vi "Pane Relief UI.vi"(8 "Error In":errorcluster, 11 "QD Launch VI Ref":refnum<vi>) -> (0 "Error Out":errorcluster)   [LabVIEW 2018]
uses:
  <resource>/dialog/QuickDrop/plugins/PaneRelief/Typedefs/Scrollbar Visibility--Enum.ctl
  <resource>/dialog/QuickDrop/plugins/PaneRelief/Typedefs/Splitter Sizing--Enum.ctl
  <resource>/dialog/QuickDrop/plugins/PaneRelief/Typedefs/Point--Cluster.ctl
  <resource>/dialog/QuickDrop/plugins/PaneRelief/Typedefs/UI Selections--Cluster.ctl
  <vilib>/Utility/sysdir.llb/System Directory Type.ctl
  <resource>/dialog/QuickDrop/plugins/PaneRelief/Classes/Splitter/Splitter.lvclass
  <resource>/dialog/QuickDrop/plugins/PaneRelief/Classes/Pane/Pane.lvclass
  <vilib>/Utility/miscctls.llb/LVRectTypeDef.ctl
  <resource>/dialog/QuickDrop/plugins/PaneRelief/Typedefs/Selection Colors--Cluster.ctl
panel:
  out "Nav Pic":picture
  in  "Label":string
  in  "Apply All - Scrollbar":bool
  in  "Apply All - Locked":bool
  in  "Apply All - Color":bool
  in  "Position":i32
  in  "Color":u32(colorbox)
  in  "Locked":bool
  in  "Sizing":T1
  in  "Vertical Scroll":T2
  in  "Horizontal Scroll":T2 caption="Scrollbar"
  in  "Origin":T3
  in  "Min Pane Size":T3
  # "Apply To All"
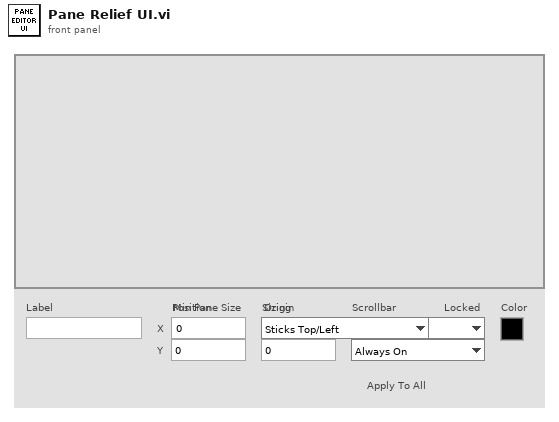
[diagram p1: front panel]
types:
  T1 = typedef "Splitter Sizing--Enum.ctl" = enum16{"Sticks Top/Left", "Sticks Bottom/Right", "Proportional"}
  T2 = typedef "Scrollbar Visibility--Enum.ctl" = enum16{"Always On", "Always Off", "Off While Running"}
  T3 = typedef "Point--Cluster.ctl" = cluster{"Horizontal":i32, "Vertical":i32}
  T4 = enum32{"Invalid", "Standard", "Closed", "Hidden", "Minimized", "Maximized"}
  T5 = enum32{"invalid app kind", "Development System", "Run Time System", "Student Edition", "Embedded LabVIEW", "Evaluation", "Custom"}
  T6 = enum16{"open", "replace", "create", "open or create", "replace or create", "replace or create with confirmation"}
  T7 = typedef "LVRectTypeDef.ctl" = cluster{"Left":i16, "Top":i16, "Right":i16, "Bottom":i16}
  T8 = typedef "LVPoint32TypeDef.ctl" = cluster{"Horizontal":i32, "Vertical":i32}
  T9 = typedef "UI Selections--Cluster.ctl" = cluster{"Mouse-over Idx":i32, "Mouse-over Splitter? (F: Pane)":bool, "Selected Idx":i32, "Selected Splitter? (F: Pane)":bool}
  T10 = cluster{"Core":cluster{"Current VI Reference":refnum<vi>, "Close Panel on Exit?":bool}, "QD Launch VI Ref":refnum<vi>, "Splitters[]":refnum<class "Splitter.lvclass">[], "Panes[]":refnum<class "Pane.lvclass">[], "UI Selections":T9, "Scale Factor":dbl, "Nav Pic Offset":T3, "Persistent Data Folder":path, "Persistent Data File":string}
  T11 = typedef "System Directory Type.ctl" = i32
  T12 = cluster{"Current VI Reference":refnum<vi>, "Close Panel on Exit?":bool}
  T13 = typedef "LVBoundsTypeDef.ctl" = cluster{"Width":u32, "Height":u32}
  T14 = typedef "LVPointTypeDef.ctl" = cluster{"Horizontal":i16, "Vertical":i16}
  T15 = typedef "Selection Colors--Cluster.ctl" = cluster{"Normal":u32, "Mouse-over":u32, "Selected":u32}
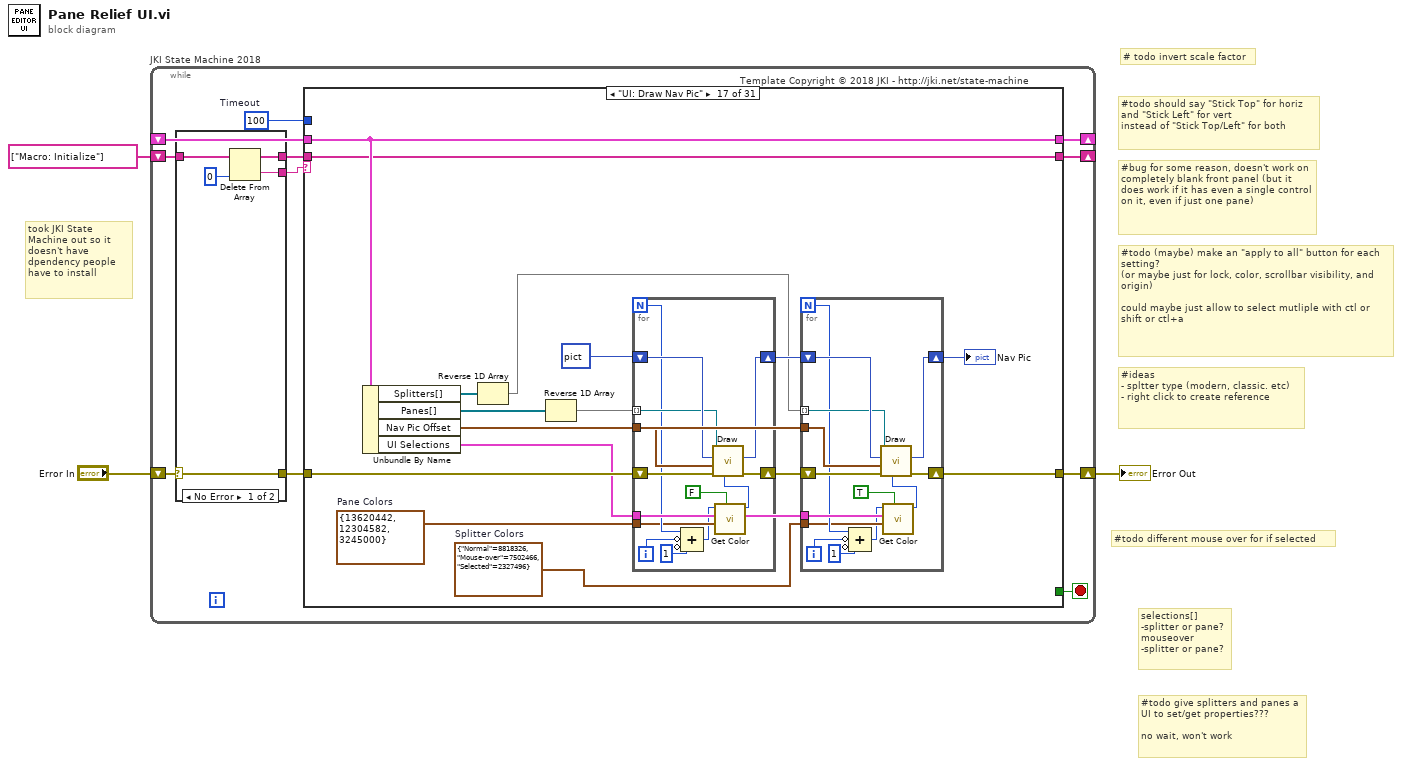
[diagram p0: block diagram]
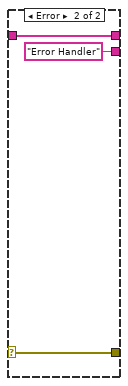
[diagram p2: hidden frame]
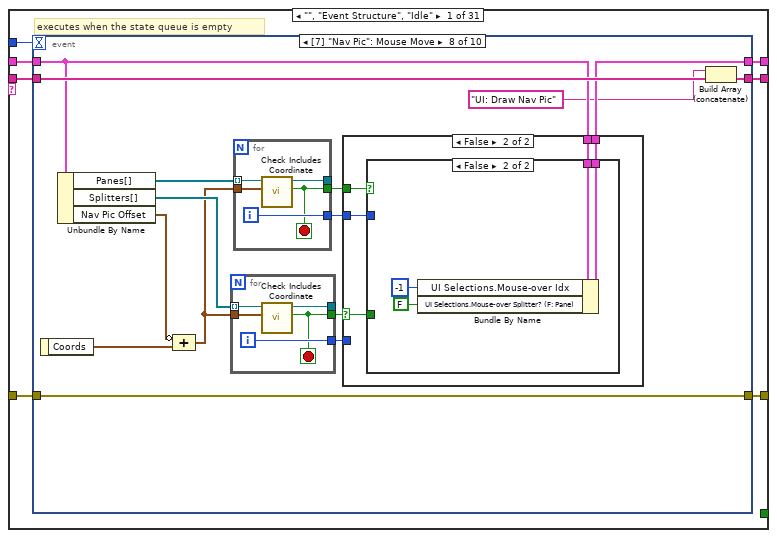
[diagram p3: hidden frame]
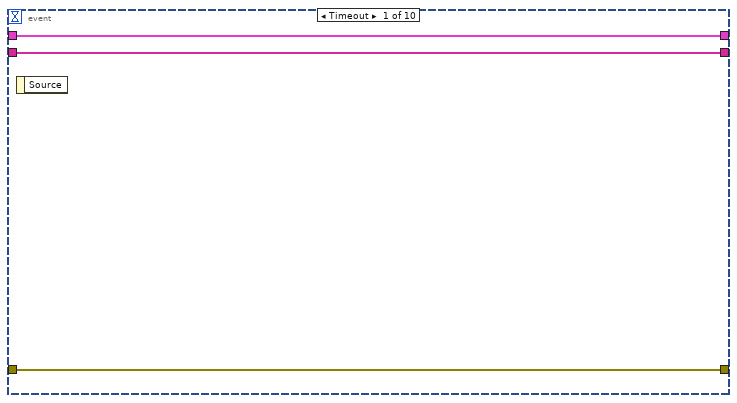
[diagram p4: hidden frame]
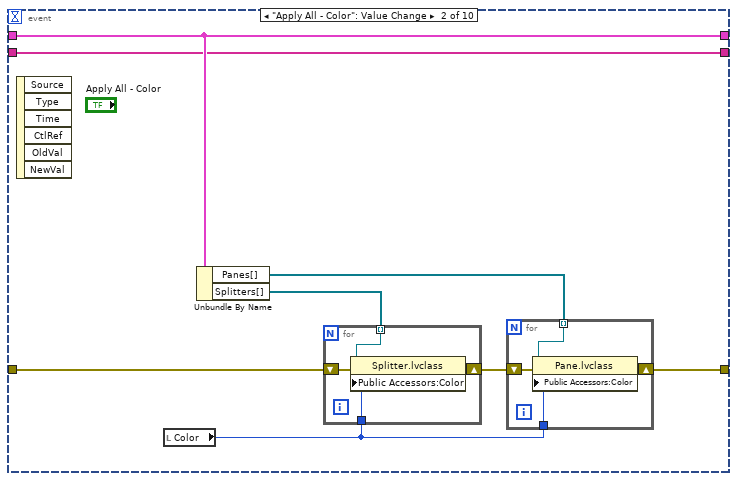
[diagram p5: hidden frame]
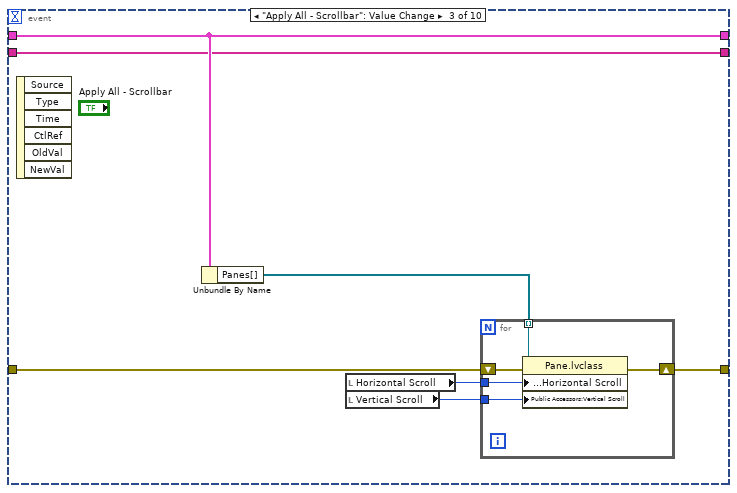
[diagram p6: hidden frame]
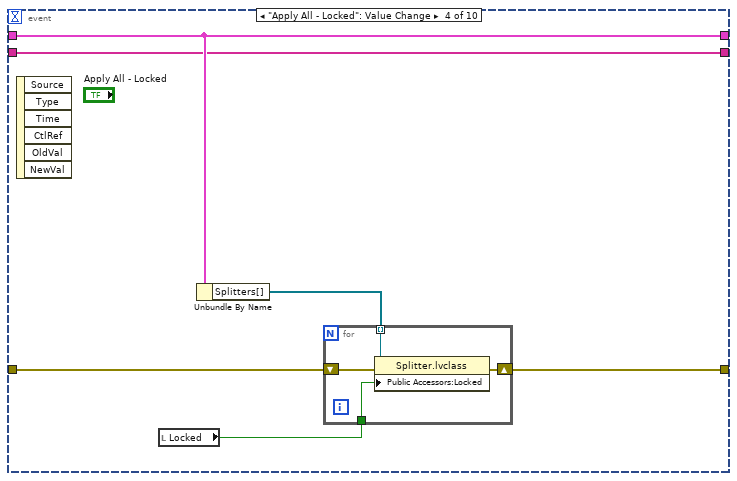
[diagram p7: hidden frame]
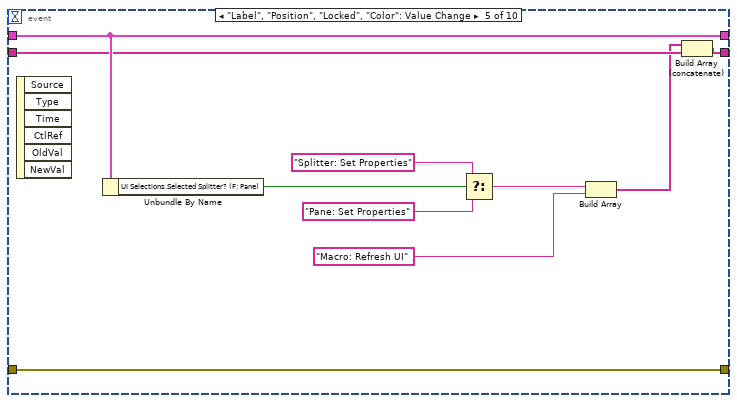
[diagram p8: hidden frame]
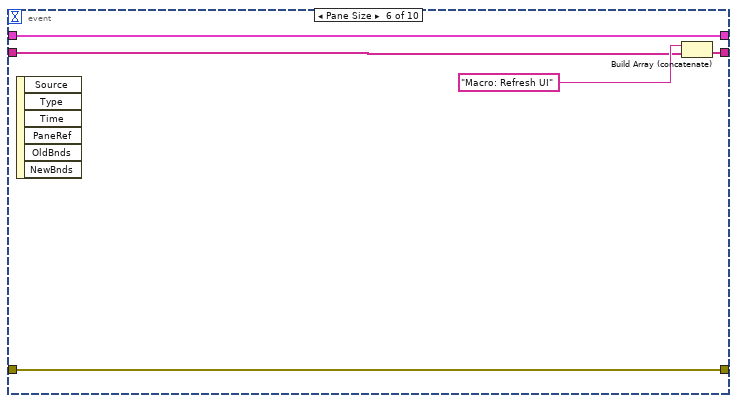
[diagram p9: hidden frame]
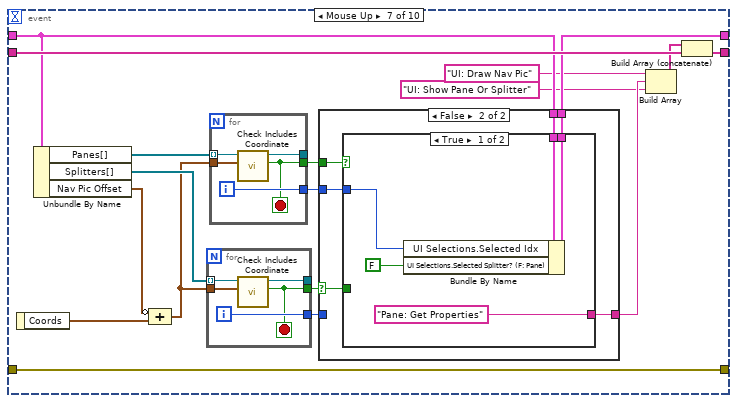
[diagram p10: hidden frame]
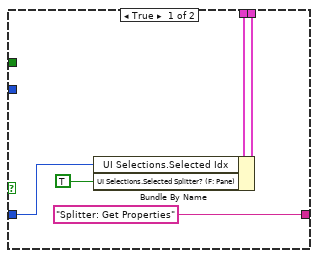
[diagram p11: hidden frame]
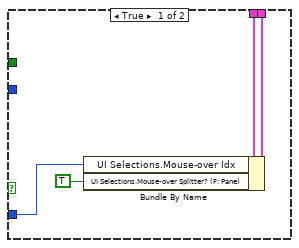
[diagram p13: hidden frame]
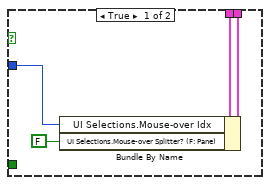
[diagram p14: hidden frame]
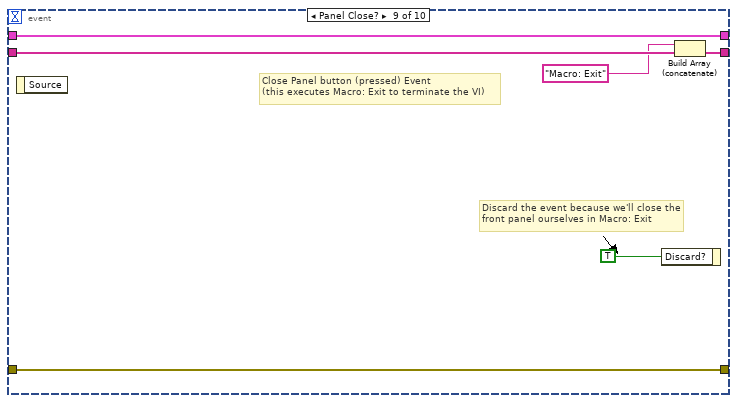
[diagram p15: hidden frame]
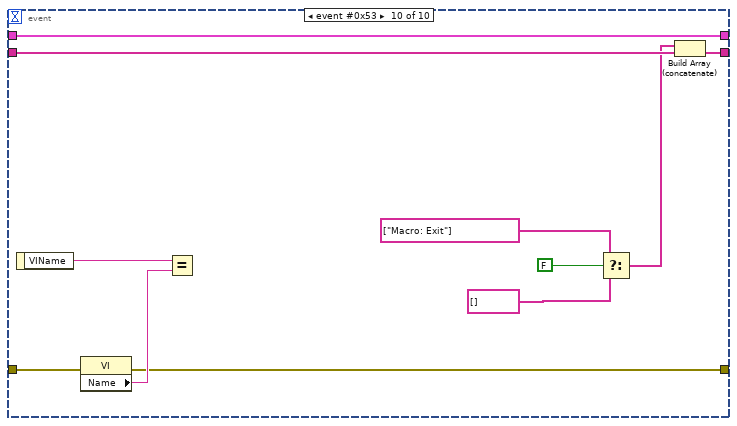
[diagram p16: hidden frame]
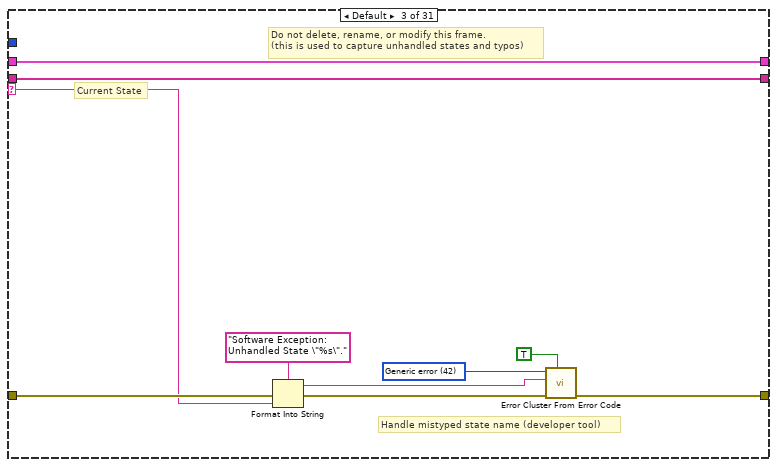
[diagram p18: hidden frame]
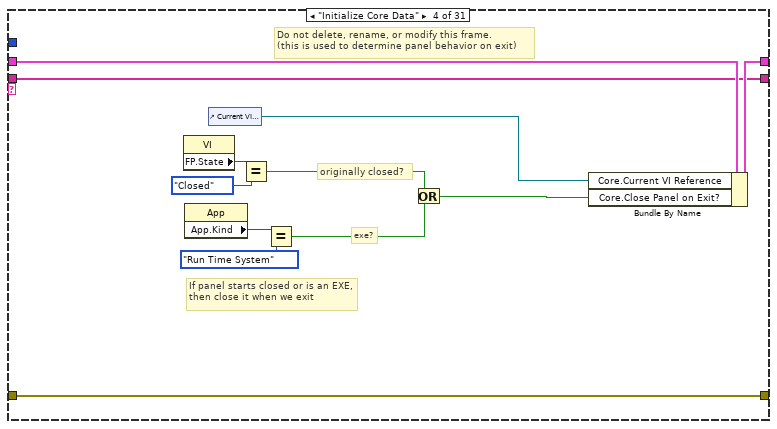
[diagram p19: hidden frame]
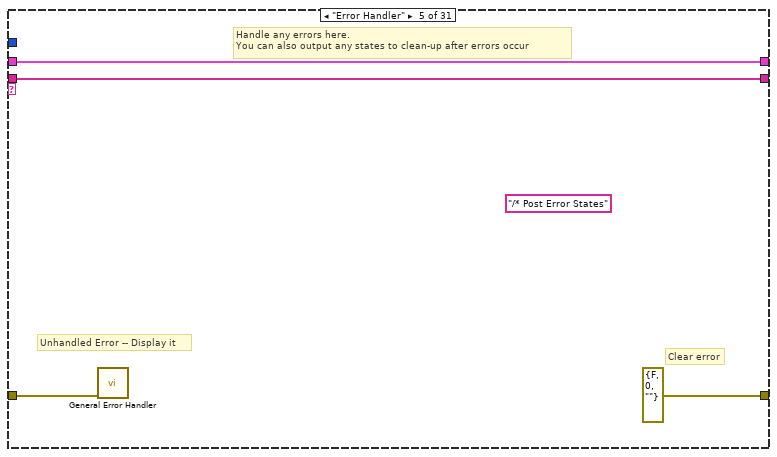
[diagram p20: hidden frame]
diagram:
  # "#todo give splitters and panes a UI to set/get properties???\n\nno wait, won't work"
  # "# todo invert scale factor"
  # "selections[]\n-splitter or pane?\nmouseover\n-splitter or pane?"
  # "#todo different mouse over for if selected"
  # "took JKI State Machine out so it doesn't have dpendency people have to install"
  # "#ideas\n- spltter type (modern, classic. etc)\n- right click to create reference"
  # "#todo (maybe) make an \"apply to all\" button for each setting?\n(or maybe just for lock, color, scrollbar visibility, and origin)\n\ncould maybe just allow to select mutliple with ctl or shift or ctl+a"
  # "#todo should say \"Stick Top\" for horiz and \"Stick Left\" for vert\ninstead of \"Stick Top/Left\" for both"
  # "#bug for some reason, doesn't work on completely blank front panel (but it does work if it has even a single control on it, even if just one pane)"
  n1 = while "JKI State Machine 2018" {
    shift-right: [w11] -> _
    shift-left: _ -> [w10]
    shift-right: [w14] -> w2
    shift-left: "Error In" -> [w4]
    shift-right: [w13] -> _
    shift-left: string[] ["Macro: Initialize"] -> [w8]
    stop <- w12 stop-if-true
    w9 = 100  # Timeout
    # "Template Copyright © 2018 JKI - http://jki.net/state-machine"
    n2 = case shown="No Error" w4 {
      selector: w4 -> [w15 w22]
      tunnel: w8 -> [w19 w21]
      tunnel: [w18 w21] -> w7
      tunnel: [w17 "Error Handler" ("String")] -> w6
      tunnel: [w15 w22] -> w5
      frame No Error {
        n3 = Delete From Array(array=w19, index=0) -> (deleted portion=w17:string, array with subset deleted=w18:string[])  [unwired: 1 in]
      }
      frame Error {
      }
    }
    n4 = case shown="\"UI: Draw Nav Pic\"" w6 {
      selector: w6 -> [_ _ w196 _ _ _ _ _ _ _ _ _ _ _ _ _ _ _ _ _ _ _ _ _ _ _ _ _ _ _ _]
      tunnel: w7 -> [w29 w190 w193 w203 w215 w219 w223 w228 w243 w248 w251 w254 w286 w311 w319 w347 w382 w412 w416 w425 w441 w450 w455 w460 w466 w473 w477 w488 w500 w503 w516]
      tunnel: w10 -> [w27 w191 w197 w209 w217 w222 w224 _ w244 w249 w253 w257 w299 w318 w326 w351 w383 w415 w419 w427 w443 w451 w456 w461 w471 w474 w487 w499 w501 w515 w528]
      tunnel: [w26 w192 w199 w213 errorcluster {"status"=FALSE, "code"=0, "source"=""} ("error out") w221 w225 w241 w245 w250 w252 w259 w287 w317 w323 w350 w374 w413 w417 w428 w444 w452 w457 w462 w472 w475 w482 w494 w502 w510 w523] -> w14
      tunnel: w5 -> [w23 w192 w198 w213 w216 w221 w225 w241 w246 w250 w252 w279 w296 w317 w331 w353 w380 w414 w418 w429 w445 w452 w457 w462 w472 w475 w483 w495 w502 w511 w524]
      tunnel: [w28 w190 w193 w203 w215 w219 w223 w228 w243 w248 w251 w254 w286 w311 w319 w347 w382 w412 w416 w425 w441 w450 w453 w458 w465 w473 w477 w488 w500 w503 w516] -> w13
      tunnel: [_ _ _ _ _ TRUE _ _ _ _ _ _ _ _ _ _ _ _ _ _ _ _ _ _ _ _ _ _ _ _ _] -> w12
      tunnel: [w25 w191 w197 w214 w217 w222 w224 w242 w244 w249 w253 w257 w299 w318 w321 w352 w383 w415 w419 w427 w443 w451 w456 w461 w471 w474 w487 w499 w501 w515 w528] -> w11
      tunnel: w9 -> [w24 _ _ _ _ _ _ _ _ _ _ _ _ _ _ _ _ _ _ _ _ _ _ _ _ _ _ _ _ _ _]
      frame "", "Event Structure", "Idle" {
        # "executes when the state queue is empty"
        n5 = event shown="[7] \"Nav Pic\": Mouse Move" {
          selector: _ -> [_ _ _ _ _ _ _ _ _ _]
          dyn-events: _ -> [_ _ _ _ _ _ _ _ _ _]
          timeout: w24 -> [_ _ _ _ _ _ _ _ _ _]
          tunnel: w29 -> [w30 w33 w49 w61 w73 w82 w103 w145 w175 w188]
          tunnel: [w30 w33 w49 w61 w71 w81 w102 w144 w173 w187] -> w28
          tunnel: w27 -> [w31 w36 w54 w64 w77 w84 w99 w141 w177 w189]
          tunnel: [w32 w37 w55 w62 w80 w85 w101 w143 w178 w184] -> w26
          tunnel: [w31 w36 w54 w64 w77 w84 w100 w142 w177 w189] -> w25
          tunnel: w23 -> [w32 w40 w52 w66 w80 w85 w101 w143 w178 w183]
          event Timeout {
            n6 = event-data() -> ()  [unwired: 1 in, 1 out]
          }
          event "Apply All - Color": Value Change {
            n7 = event-data() -> ()  [unwired: 1 in, 6 out]
            n8 = local read "Color"() -> (w38:u32)
            n9 = Unbundle By Name(w36) -> ("Panes[]"=w34:refnum<class "Pane.lvclass">[], "Splitters[]"=w35:refnum<class "Splitter.lvclass">[])
            n10 = for {
              tunnel: w38 -> [w45]
              shift-right: [w47] -> w39
              shift-left: w40 -> [w48]
              tunnel: w35 -> [w46] mode=indexing
              n11 = property class="Splitter.lvclass"(reference=w46, error in=w48, "Public Accessors:Color"=w45) -> (error out=w47:errorcluster)  [unwired: 1 out]
            }
            n12 = for {
              tunnel: w38 -> [w43]
              shift-right: [w42] -> w37
              shift-left: w39 -> [w44]
              tunnel: w34 -> [w41] mode=indexing
              n13 = property class="Pane.lvclass"(reference=w41, error in=w44, "Public Accessors:Color"=w43) -> (error out=w42:errorcluster)  [unwired: 1 out]
            }
          }
          event "Apply All - Scrollbar": Value Change {
            n14 = event-data() -> ()  [unwired: 1 in, 6 out]
            n15 = Unbundle By Name(w54) -> ("Panes[]"=w53:refnum<class "Pane.lvclass">[])
            n16 = local read "Horizontal Scroll"() -> (w51:T2)
            n17 = local read "Vertical Scroll"() -> (w50:T2)
            n18 = for {
              shift-right: [w59] -> w55
              shift-left: w52 -> [w60]
              tunnel: w53 -> [w58] mode=indexing
              tunnel: w51 -> [w57]
              tunnel: w50 -> [w56]
              n19 = property class="Pane.lvclass"(reference=w58, error in=w60, "Public Accessors:Horizontal Scroll"=w57, "Public Accessors:Vertical Scroll"=w56) -> (error out=w59:errorcluster)  [unwired: 1 out]
            }
          }
          event "Apply All - Locked": Value Change {
            n20 = event-data() -> ()  [unwired: 1 in, 6 out]
            n21 = local read "Locked"() -> (w65:bool)
            n22 = Unbundle By Name(w64) -> ("Splitters[]"=w63:refnum<class "Splitter.lvclass">[])
            n23 = for {
              tunnel: w65 -> [w68]
              shift-right: [w69] -> w62
              shift-left: w66 -> [w70]
              tunnel: w63 -> [w67] mode=indexing
              n24 = property class="Splitter.lvclass"(reference=w67, error in=w70, "Public Accessors:Locked"=w68) -> (error out=w69:errorcluster)  [unwired: 1 out]
            }
          }
          event "Label", "Position", "Locked", "Color": Value Change {
            n25 = event-data() -> ()  [unwired: 1 in, 6 out]
            n26 = Unbundle By Name(w77) -> ("UI Selections.Selected Splitter? (F: Pane)"=w76:bool)
            n27 = Select(t="Splitter: Set Properties" ("State(s) in Front (\"\")"), s=w76, f="Pane: Set Properties" ("State(s) in Front (\"\")")) -> (s? t:f=w75:string)
            n28 = Build Array(w75, "Macro: Refresh UI" ("State(s) in Front (\"\")")) -> (w72:string[])
            n29 = Build Array (concatenate)(w72, w73) -> (w71:string[])
          }
          event Pane Size {
            n30 = event-data() -> ()  [unwired: 1 in, 6 out]
            n31 = Build Array (concatenate)("Macro: Refresh UI", w82) -> (w81:string[])
          }
          event Mouse Up {
            n32 = event-data() -> ("Coords"=w92:T8)  [unwired: 1 in]
            n33 = Unbundle By Name(w99) -> ("Panes[]"=w90:refnum<class "Pane.lvclass">[], "Splitters[]"=w89:refnum<class "Splitter.lvclass">[], "Nav Pic Offset"=w93:T3)
            n34 = Compound Arithmetic op=ADD(invert w93, w92) -> (w88:T3)
            n35 = for {
              tunnel: [w108] -> _
              tunnel: [w104] -> w98
              tunnel: w89 -> [w107] mode=indexing
              tunnel: w88 -> [w106]
              tunnel: [w105] -> w86
              i -> [w105]
              stop <- w104 stop-if-true
              n36 = call-dynamic "Check Includes Coordinate.vi"("Coordinate"=w106, "Panel Object in"=w107) -> ("Included?"=w104:bool, "Panel Object out"=w108:refnum<class "Splitter.lvclass">)  [unwired: 7 in, 1 out]
            }
            n37 = for {
              tunnel: [w109] -> w97
              tunnel: [w113] -> _
              tunnel: w90 -> [w112] mode=indexing
              tunnel: w88 -> [w111]
              tunnel: [w110] -> w87
              i -> [w110]
              stop <- w109 stop-if-true
              n38 = call-dynamic "Check Includes Coordinate.vi"("Coordinate"=w111, "Panel Object in"=w112) -> ("Included?"=w109:bool, "Panel Object out"=w113:refnum<class "Pane.lvclass">)  [unwired: 7 in, 1 out]
            }
            n39 = case shown="False" w98 {
              selector: w98 -> [_ w122]
              tunnel: [w118 w124] -> w100
              tunnel: w99 -> [w117 w123]
              tunnel: w97 -> [_ w121]
              tunnel: ["Splitter: Get Properties" w120] -> w96
              tunnel: w87 -> [_ w119]
              tunnel: w86 -> [w114 _]
              frame True {
                n40 = Bundle By Name(cluster=w117, "UI Selections.Selected Idx"=w114, "UI Selections.Selected Splitter? (F: Pane)"=TRUE ("UI Selections.Splitter? (F: Pane)")) -> (w118:T10)
              }
              frame False {
                n41 = case shown="True" w121 {
                  tunnel: [w129 w130] -> w124
                  tunnel: w123 -> [w128 w130]
                  tunnel: w122 -> [_ _]
                  tunnel: ["Pane: Get Properties" _] -> w120
                  tunnel: w119 -> [w125 _]
                  frame True {
                    n42 = Bundle By Name(cluster=w128, "UI Selections.Selected Idx"=w125, "UI Selections.Selected Splitter? (F: Pane)"=FALSE ("UI Selections.Splitter? (F: Pane)")) -> (w129:T10)
                  }
                  frame False {
                  }
                }
              }
            }
            n43 = Build Array("UI: Draw Nav Pic", w96, "UI: Show Pane Or Splitter") -> (w94:string[])
            n44 = Build Array (concatenate)(w94, w103) -> (w102:string[])
          }
          event "Nav Pic": Mouse Move {
            n45 = event-data() -> ("Coords"=w137:T8)  [unwired: 1 in]
            n46 = Unbundle By Name(w141) -> ("Panes[]"=w136:refnum<class "Pane.lvclass">[], "Splitters[]"=w135:refnum<class "Splitter.lvclass">[], "Nav Pic Offset"=w138:T3)
            n47 = Compound Arithmetic op=ADD(invert w138, w137) -> (w134:T3)
            n48 = for {
              tunnel: [w150] -> _
              tunnel: [w146] -> w140
              tunnel: w135 -> [w149] mode=indexing
              tunnel: w134 -> [w148]
              tunnel: [w147] -> w132
              i -> [w147]
              stop <- w146 stop-if-true
              n49 = call-dynamic "Check Includes Coordinate.vi"("Coordinate"=w148, "Panel Object in"=w149) -> ("Included?"=w146:bool, "Panel Object out"=w150:refnum<class "Splitter.lvclass">)  [unwired: 7 in, 1 out]
            }
            n50 = for {
              tunnel: [w151] -> w139
              tunnel: [w155] -> _
              tunnel: w136 -> [w154] mode=indexing
              tunnel: w134 -> [w153]
              tunnel: [w152] -> w133
              i -> [w152]
              stop <- w151 stop-if-true
              n51 = call-dynamic "Check Includes Coordinate.vi"("Coordinate"=w153, "Panel Object in"=w154) -> ("Included?"=w151:bool, "Panel Object out"=w155:refnum<class "Pane.lvclass">)  [unwired: 7 in, 1 out]
            }
            n52 = case shown="False" w140 {
              selector: w140 -> [_ w162]
              tunnel: [w159 w164] -> w142
              tunnel: w141 -> [w158 w163]
              tunnel: w139 -> [_ w161]
              tunnel: w133 -> [_ w160]
              tunnel: w132 -> [w156 _]
              frame True {
                n53 = Bundle By Name(cluster=w158, "UI Selections.Mouse-over Idx"=w156, "UI Selections.Mouse-over Splitter? (F: Pane)"=TRUE ("UI Selections.Splitter? (F: Pane)")) -> (w159:T10)
              }
              frame False {
                n54 = case shown="False" w161 {
                  tunnel: [w168 w169] -> w164
                  tunnel: w163 -> [w167 w170]
                  tunnel: w162 -> [_ _]
                  tunnel: w160 -> [w165 _]
                  frame True {
                    n55 = Bundle By Name(cluster=w167, "UI Selections.Mouse-over Idx"=w165, "UI Selections.Mouse-over Splitter? (F: Pane)"=FALSE ("UI Selections.Splitter? (F: Pane)")) -> (w168:T10)
                  }
                  frame False {
                    n56 = Bundle By Name(cluster=w170, "UI Selections.Mouse-over Idx"=-1, "UI Selections.Mouse-over Splitter? (F: Pane)"=FALSE ("UI Selections.Splitter? (F: Pane)")) -> (w169:T10)
                  }
                }
              }
            }
            n57 = Build Array (concatenate)("UI: Draw Nav Pic", w145) -> (w144:string[])
          }
          event Panel Close? {
            # "Discard the event because we'll close the front panel ourselves in Macro: Exit"
            # "Close Panel button (pressed) Event\n(this executes Macro: Exit to terminate the VI)"
            n58 = event-data() -> ()  [unwired: 1 in, 1 out]
            n59 = event-data("Discard?"=TRUE) -> ()  [unwired: 1 in, 1 out]
            n60 = Build Array (concatenate)("Macro: Exit", w175) -> (w173:string[])
          }
          event event #0x53 {
            n61 = event-data() -> ("VIName"=w186:string)  [unwired: 1 in]
            n62 = property class="VI"(error in=w183) -> (error out=w184:errorcluster, "Name"=w185:string)  [unwired: 1 in, 1 out]
            n63 = Equal?(x=w186, y=w185) -> ()  [unwired: 1 out]
            n64 = Select(t=string[] ["Macro: Exit"], s=FALSE, f=string[] []) -> (s? t:f=w180:string[])
            n65 = Build Array (concatenate)(w180, w188) -> (w187:string[])
          }
        }
      }
      frame "---------- Core ----------" {
        # "Do not put any code in this frame.\n(it is a separator no-op)"
      }
      frame Default {
        w195 = 42 items=["No error", "Argument error", "Memory is full", "Out of zone", "End of file", "File already open", "Generic file I/O error", "File not found", "File permission error", "Disk is full", "Duplicate path", "Too many files open", "System feature not enabled", "Resource file not found", "Cannot add resource", "Resource not found", "Image not found", "Image memory error", "Pen does not exist", "Config type invalid", "Config token not found", "Config parse error", "Config memory error", "Bad external code format", "Bad external code offset", "External code not present", "Null window", "Destroy window error", "Null menu", "Print aborted", "Bad print record", "Print driver error", "Windows error during printing", "Memory error during printing", "Print dialog error", "Generic print error", "Invalid device refnum", "Device not found", "Device parameter error", "Device unit error", "Cannot open device", "Device call aborted", "Generic error", "Cancelled by user", "Object ID too low", "Object ID too high", "Object not in heap", "Unknown heap", "Unknown object (invalid DefProc)", "Unknown object (DefProc not in table)", "Message out of range", "Invalid (null) method", "Unknown message", "Manager call not supported", "Bad address", "Network operation in progress", "Network operation timed out", "Connection is busy", "Network attribute not supported", "Network error", "Address in use", "System out of memory", "Connection aborted", "Connection refused", "Not connected", "Already connected", "Connection closed", "Initialization error (interapplication manager)", "Bad occurrence", "Wait on unbound occurrence handler", "Occurrence queue overflow", "Datalog type conflict", "Unused", "Unrecognized type (interapplication manager)", "Memory corrupt", "Failed to make temporary DLL", "Old CIN version", "Drag socket not found", "Failed to load drop-object", "Failed to register OLE object", "Failed to release OLE object", "Format specifier type mismatch", "Unknown format specifier", "Too few format specifiers", "Too many format specifiers", "Scan failed", "Newer CIN version", "Error converting to variant", "Runtime menu error", "Password tampered", "Variant attribute not found", "Incompatible variant data type", "Event data is not available", "Event Store is not present", "Occurrence is not found", "Event Queue is not created", "Event info is not available", "Refnum passed is NULL", "Error retrieving Class GUID", "Error retrieving CoClass GUID", "Error retrieving TypeLib GUID.", "Bad built application magic bytes.", "Specific driver is different from the specific driver associated with the Logical Name.", "There is no session opened to the class driver.", "Max Error", "MAX - Error with config objects", "MAX - Error loading configuration", "MAX - Group not supported"]
        # "Current State"
        # "Do not delete, rename, or modify this frame.\n(this is used to capture unhandled states and typos)"
        # "Handle mistyped state name (developer tool)"
        n66 = Format Into String(format string="Software Exception: Unhandled State \"%s\"." ("message"), error in=w198, w196) -> (resulting string=w201:string, error out=w200:errorcluster)  [unwired: 1 in]
        n67 = call <vilib>:"Error Cluster From Error Code.vi"("show call chain? (False)"=TRUE, "error in (no error)"=w200, "error message (\"\")"=w201, "error code (0)"=w195) -> ("error out"=w199:errorcluster)  [unwired: 5 in]
      }
      frame "Initialize Core Data" {
        # "Do not delete, rename, or modify this frame.\n(this is used to determine panel behavior on exit)"
        # "originally closed?"
        # "exe?"
        # "If panel starts closed or is an EXE, then close it when we exit"
        n68 = property class="VI"() -> ("FP.State"=w206:T4)  [unwired: 2 in, 2 out]
        n69 = property class="App"() -> ("App.Kind"=w212:T5)  [unwired: 2 in, 2 out]
        n70 = control-ref of="Current VI Reference"() -> (w207:refnum<vi>)
        n71 = Equal?(x=w206, y=T4."Closed" ("Front Panel Window:State")) -> (x = y?=w204:bool)
        n72 = Equal?(x=w212, y=T5."Run Time System" ("Application:Kind")) -> (x = y?=w210:bool)
        n73 = Or(x=w204, y=w210) -> (x .or. y?=w208:bool)
        n74 = Bundle By Name(cluster=w209, "Core.Current VI Reference"=w207, "Core.Close Panel on Exit?"=w208) -> (w214:T10)
      }
      frame "Error Handler" {
        (unwired) "/* Post Error States"
        # "Unhandled Error -- Display it"
        # "Handle any errors here.\nYou can also output any states to clean-up after errors occur"
        # "Clear error"
        n75 = call <vilib>:"General Error Handler.vi"("error in (no error)"=w216) -> ()  [unwired: 10 in, 5 out]
      }
      frame "Exit" {
        # "Do not put any code in this frame.\n(No errors that occur here will be handled.)"
      }
      frame "---------- Data ----------" {
        # "Do not put any code in this frame.\n(It is a separator no-op. You can make a copy of this frame to create a new Data frame)"
      }
      frame "Data: Initialize" {
        w226 = refnum<class "Pane.lvclass">[] []  # Panes[]
        w227 = refnum<class "Splitter.lvclass">[] []  # Splitters[]
        w232 = path ""  # Persistent Data Folder
        w229 = "PaneReliefPersistentData.txt"  # Persistent Data File
        w235 = T11 3 items=["User Home"=0, "User Desktop"=1, "User Documents"=2, "User Application Data"=3, "User Preferences"=4, "User Temporary"=5, "Public Documents"=6, "Public Application Data"=7, "Public Preferences"=8, "Public Cache"=13, "System Core Libraries"=9, "System Installed Libraries"=10, "Application Files"=11, "Boot Volume Root"=12] ("system directory type")
        w236 = T3 {"Horizontal"=0, "Vertical"=0}  # Nav Pic Offset
        w237 = 0.0  # Scale Factor
        w238 = T9 {"Mouse-over Idx"=-1, "Mouse-over Splitter? (F: Pane)"=FALSE, "Selected Idx"=0, "Selected Splitter? (F: Pane)"=FALSE}  # UI Selections
        w239 = T12 {"Current VI Reference"=refnum, "Close Panel on Exit?"=FALSE}  # Core
        # "Data names and types of shift register data are defined by this bundle."
        # "Initialize the shift-register data, here.\n(data names are defined by what you wire into the bundle function)"
        n76 = call <vilib>:"Get System Directory.vi"("system directory type"=w235) -> ("system directory"=w233:path)  [unwired: 10 in]
        n77 = Build Path(base path=w233, name or relative path="PaneRelief") -> (appended path=w230:path)
        n78 = Variant To Data(type=w232, Variant=w230) -> (data=w231:path)  [unwired: 1 in, 1 out]
        n79 = Bundle("Core"=w239, "QD Launch VI Ref"="QD Launch VI Ref", "Splitters[]"=w227, "Panes[]"=w226, "UI Selections"=w238, "Scale Factor"=w237, "Nav Pic Offset"=w236, "Persistent Data Folder"=w231, "Persistent Data File"=w229) -> (w242:T10)  [unwired: 1 in]
      }
      frame "Data: Cleanup" {
        # "Cleanup any data and references, here.\n(this is called automatically, by the Macro: Exit)"
        n80 = Unbundle By Name(w244) -> ("Core.Current VI Reference"=w247:refnum<vi>)
        n81 = Close Reference(reference=w247, error in (no error)=w246) -> (error out=w245:errorcluster)
      }
      frame "---------- UI ----------" {
        # "Do not put any code in this frame.\n(It is a separator no-op. You can make a copy of this frame to create a new UI frame)"
      }
      frame "UI: Initialize" {
        # "Initialize the User Interface, here.\n(this is called automatically, by the Macro: Init)"
      }
      frame "UI: Save Window Bounds" {
        n82 = property class="VI"(error in=w279) -> (error out=w278:errorcluster, "Front Panel.WinBounds"=w263:T7)  [unwired: 1 in, 1 out]
        n83 = Unbundle By Name(w257) -> ("Persistent Data Folder"=w256:path, "Persistent Data File"=w255:string)
        n84 = Unbundle By Name(w263) -> ("Left"=w268:i16, "Top"=w266:i16, "Right"=w265:i16, "Bottom"=w264:i16)
        n85 = Format Into String(format string="%d,%d,%d,%d", error in=w278, w268, w266, w265, w264) -> (resulting string=w262:string, error out=w269:errorcluster)  [unwired: 1 in]
        n86 = call <vilib>:"Check if File or Folder Exists.vi"("error in (no error)"=w269, "path"=w256) -> ("error out"=w277:errorcluster, "file or folder exists?"=w276:bool, "dup path"=w275:path)  [unwired: 7 in]
        n87 = case shown="False" w276 {
          tunnel: w277 -> [w283 w284]
          tunnel: w275 -> [w282 w285]
          tunnel: [w281 w285] -> w273
          tunnel: [w280 w284] -> w271
          frame False {
            n88 = Create Folder(path (use dialog)=w282, error in=w283) -> (created path=w281:path, error out=w280:errorcluster)  [unwired: 1 in, 1 out]
          }
          frame True {
          }
        }
        n89 = Build Path(base path=w273, name or relative path=w255) -> (appended path=w272:path)
        n90 = Open/Create/Replace File(file path (use dialog)=w272, error in=w271, operation (0:open)=T6."replace or create") -> (refnum out=w274:refnum<file>, error out=w270:errorcluster)  [unwired: 3 in, 1 out]
        n91 = Write to Text File(file (use dialog)=w274, text=w262, error in=w270) -> (refnum out=w258:refnum<file>, error out=w260:errorcluster)  [unwired: 1 in, 1 out]
        n92 = Close File(refnum=w258, error in=w260) -> (error out=w259:errorcluster)  [unwired: 1 out]
      }
      frame "UI: Load Window Bounds" {
        n93 = Unbundle By Name(w299) -> ("Persistent Data Folder"=w298:path, "Persistent Data File"=w297:string)
        n94 = Build Path(base path=w298, name or relative path=w297) -> (appended path=w300:path)
        n95 = Read from Text File(file (use dialog)=w300, error in=w296) -> (text=w293:string, error out=w295:errorcluster)  [unwired: 2 in, 2 out]
        n96 = Scan From String(format string="%d,%d,%d,%d", input string=w293, error in=w295) -> (error out=w288:errorcluster, output 1=w292:i32, output 2=w291:i32, output 3=w290:i32, output 4=w289:i32)  [unwired: 5 in, 2 out]
        n97 = case shown="No Error" w288 {
          selector: w288 -> [w302 w310]
          tunnel: w292 -> [w307 _]
          tunnel: w291 -> [w306 _]
          tunnel: w290 -> [w305 _]
          tunnel: w289 -> [w304 _]
          tunnel: [w301 w309] -> w287
          frame No Error {
            n98 = Bundle By Name(cluster=T7 {"Left"=0, "Top"=0, "Right"=0, "Bottom"=0} ("Front Panel Window:Window Bounds"), "Left"=w307, "Top"=w306, "Right"=w305, "Bottom"=w304) -> (w303:T7)
            n99 = property class="VI"(error in=w302, "Front Panel.WinBounds"=w303) -> (error out=w301:errorcluster)  [unwired: 1 in, 1 out]
          }
          frame Error {
            # "first time running or persistent data file was deleted, no problem, just can't restore previous window position"
            n100 = call <vilib>:"Clear Errors.vi"("error in (no error)"=w310) -> ("error out"=w309:errorcluster)  [unwired: 5 in, 1 out]
          }
        }
      }
      frame "UI: Show Pane Or Splitter" {
        # "Splitter-specific controls"
        # "Pane-specific controls"
        n101 = Unbundle By Name(w318) -> ("UI Selections.Selected Idx"=w316:i32, "UI Selections.Selected Splitter? (F: Pane)"=w314:bool)
        n102 = Greater Or Equal To 0?(x=w316) -> (x >= 0?=w315:bool)
        n103 = Compound Arithmetic op=AND(w315, invert w314) -> (w312:bool)
        n104 = Compound Arithmetic op=AND(w315, w314) -> (w313:bool)
        n105 = property on="Position" class="DigNum (strict)"("Visible"=w313) -> ()  [unwired: 2 in, 2 out]
        n106 = property on="Sizing" class="Enum (strict)"("Visible"=w313) -> ()  [unwired: 2 in, 2 out]
        n107 = property on="Locked" class="Bool (strict)"("Visible"=w313) -> ()  [unwired: 2 in, 2 out]
        n108 = property on="Apply All - Locked" class="Bool"("Visible"=w313) -> ()  [unwired: 2 in, 2 out]
        n109 = property on="Min Pane Size" class="Clust (strict)"("Visible"=w312) -> ()  [unwired: 2 in, 2 out]
        n110 = property on="Origin" class="Clust (strict)"("Visible"=w312) -> ()  [unwired: 2 in, 2 out]
        n111 = property on="Horizontal Scroll" class="Enum (strict)"("Visible"=w312) -> ()  [unwired: 2 in, 2 out]
        n112 = property on="Vertical Scroll" class="Enum (strict)"("Visible"=w312) -> ()  [unwired: 2 in, 2 out]
        n113 = property on="Apply All - Scrollbar" class="Bool"("Visible"=w312) -> ()  [unwired: 2 in, 2 out]
      }
      frame "UI: Calculate Scale Factor" {
        # "#todo doesn't give right area if VI is empty"
        n114 = Unbundle By Name(w326) -> ("QD Launch VI Ref"=w329:refnum<vi>)
        n115 = property class="VI"(reference=w329, error in=w331) -> (error out=w333:errorcluster, "Panel"=w332:refnum<vi>)  [unwired: 1 out]
        n116 = property class="Pnl"(reference=w332, error in=w333) -> (error out=w328:errorcluster, "Width"=w330:u32, "Height"=w334:u32)  [unwired: 1 out]
        n117 = property on="Nav Pic" class="Pict"(error in=w328) -> (error out=w323:errorcluster, "Draw Area Size"=w327:T13)  [unwired: 1 in, 1 out]
        n118 = Unbundle By Name(w327) -> ("Width"=w325:u32, "Height"=w324:u32)
        n119 = call <resource>:"Calculate Scaling Factors.vi"("Max Picture Size Y"=w324, "Max Picture Size X"=w325, "Panel Height"=w334, "Panel Width"=w330) -> ("Scale Factor"=w322:dbl, "Offset (to center)"=w320:T3)  [unwired: 6 in]
        n120 = Bundle By Name(cluster=w326, "Nav Pic Offset"=w320, "Scale Factor"=w322) -> (w321:T10)
      }
      frame "UI: Get Pane And Splitter Details" {
        n121 = Unbundle By Name(w351) -> ("Scale Factor"=w348:dbl, "QD Launch VI Ref"=w341:refnum<vi>)
        n122 = property class="VI"(reference=w341, error in=w353) -> (error out=w355:errorcluster, "Panel"=w354:refnum<vi>)  [unwired: 1 out]
        n123 = property class="Pnl"(reference=w354, error in=w355) -> (error out=w338:errorcluster, "Panes[]"=w340:refnum<vi>[], "Splitters[]"=w342:refnum<vi>[])  [unwired: 1 out]
        n124 = Index Array(array=w340) -> (element=w335:refnum<vi>)  [unwired: 1 in]
        n125 = property class="Pane"(reference=w335, error in=w338) -> (reference out=w346:refnum<vi>, error out=w345:errorcluster, "Origin"=w344:T14)
        n126 = invoke on="Invoke Node" class="Pane" method="CvtPaneToPanelCoords"(reference=w346, error in=w345, "PaneCoords"=w344) -> (error out=w337:errorcluster, "PanelCoords"=w336:T14)  [unwired: 2 in, 3 out]
        n127 = for {
          tunnel: w348 -> [w365]
          tunnel: w340 -> [w364] mode=indexing
          shift-right: [w366] -> w349
          shift-left: w337 -> [w367]
          tunnel: [w363] -> w343 mode=indexing
          tunnel: w336 -> [w362]
          n128 = call <resource>:"Pane.vi"("Error In"=w367, "Offset"=w362, "Scale Factor"=w365, "Pane Ref"=w364) -> ("Error Out"=w366:errorcluster, "Pane out"=w363:refnum<class "Pane.lvclass">)  [unwired: 6 in]
        }
        n129 = for {
          tunnel: w348 -> [w359]
          tunnel: w342 -> [w358] mode=indexing
          shift-right: [w361] -> w350
          shift-left: w349 -> [w360]
          tunnel: [w357] -> w339 mode=indexing
          tunnel: w336 -> [w356]
          n130 = call <resource>:"Splitter.vi"("Error In"=w360, "Offset"=w356, "Scale Factor"=w359, "Splitter Ref"=w358) -> ("Error Out"=w361:errorcluster, "Splitter out"=w357:refnum<class "Splitter.lvclass">)  [unwired: 6 in]
        }
        n131 = Bundle By Name(cluster=w351, "Panes[]"=w343, "Splitters[]"=w339) -> (w352:T10)
      }
      frame "UI: Draw Nav Pic" {
        w368 = T15 {"Normal"=8818326, "Mouse-over"=7502466, "Selected"=2327496}  # Splitter Colors
        w369 = T15 {"Normal"=13620442, "Mouse-over"=12304582, "Selected"=3245000}  # Pane Colors
        n132 = Unbundle By Name(w383) -> ("Splitters[]"=w379:refnum<class "Splitter.lvclass">[], "Panes[]"=w378:refnum<class "Pane.lvclass">[], "Nav Pic Offset"=w370:T3, "UI Selections"=w372:T9)
        n133 = Reverse 1D Array(array=w379) -> (reversed array=w371:refnum<class "Splitter.lvclass">[])
        n134 = Reverse 1D Array(array=w378) -> (reversed array=w377:refnum<class "Pane.lvclass">[])
        n135 = for {
          N -> [w404]
          shift-right: [w411] -> w376
          shift-left: picture data[5B] ("Picture out") -> [w410]
          tunnel: w370 -> [w409]
          shift-right: [w407] -> w373
          shift-left: w380 -> [w408]
          tunnel: w372 -> [w406]
          tunnel: w377 -> [w405] mode=indexing
          tunnel: w369 -> [w400]
          i -> [w403]
          n136 = Compound Arithmetic op=ADD(w404, invert w403, invert 1 ("value")) -> (w399:i32)
          n137 = call <resource>:"Get Color.vi"("Splitter? (F: Pane)"=FALSE, "Pane Colors"=w400, "UI Selections"=w406, "Item Index"=w399) -> ("Color"=w402:u32)  [unwired: 7 in]
          n138 = call-dynamic "Draw.vi"("Color Box"=w402, "Error In"=w408, "Offset"=w409, "Picture in"=w410, "Panel Object in"=w405) -> ("Error Out"=w407:errorcluster, "Picture out"=w411:picture)  [unwired: 4 in, 1 out]
        }
        n139 = for {
          N -> [w390]
          shift-right: [w397] -> w375
          shift-left: w376 -> [w396]
          tunnel: w370 -> [w395]
          shift-right: [w393] -> w374
          shift-left: w373 -> [w394]
          tunnel: w372 -> [w392]
          tunnel: w371 -> [w391] mode=indexing
          tunnel: w368 -> [w386]
          i -> [w389]
          n140 = Compound Arithmetic op=ADD(w390, invert w389, invert 1 ("value")) -> (w385:i32)
          n141 = call <resource>:"Get Color.vi"("Splitter? (F: Pane)"=TRUE, "Pane Colors"=w386, "UI Selections"=w392, "Item Index"=w385) -> ("Color"=w388:u32)  [unwired: 7 in]
          n142 = call-dynamic "Draw.vi"("Color Box"=w388, "Error In"=w394, "Offset"=w395, "Picture in"=w396, "Panel Object in"=w391) -> ("Error Out"=w393:errorcluster, "Picture out"=w397:picture)  [unwired: 4 in, 1 out]
        }
        "Nav Pic" <- w375
      }
      frame "UI: Cursor Set >> Idle" {
        # "Argument"
        # "Set and Unset Cursor Busy.\n(Usage: \"UI: Cursor Set >> Busy|Idle\")"
        n143 = call <vilib>:"Unset Busy.vi"("error in (no error)"=w414) -> ("error out"=w413:errorcluster)  [unwired: 10 in]
      }
      frame "UI: Cursot Set >> Busy" {
        # "Argument"
        # "Set and Unset Cursor Busy.\n(Usage: \"UI: Cursor Set >> Busy|Idle\")"
        n144 = call <vilib>:"Set Busy.vi"("error in (no error)"=w418) -> ("error out"=w417:errorcluster)  [unwired: 9 in, 1 out]
      }
      frame "UI: Front Panel State >> Open" {
        w420 = T4."Standard" ("State")
        # "Set Front Panel Open or Closed\n(Usage: \"UI: Front Panel State >> Open|Close\")"
        n145 = Unbundle By Name(w427) -> ("Core.Current VI Reference"=w426:refnum<vi>)
        n146 = property class="VI"(reference=w426, error in=w429) -> (reference out=w423:refnum<vi>, error out=w424:errorcluster, "FP.State"=w422:T4)
        n147 = Not Equal?(x=w422, y=w420) -> (x != y?=w421:bool)
        n148 = case shown="True" w421 {
          tunnel: [w433 w435] -> w428
          tunnel: w424 -> [w432 w435]
          tunnel: w423 -> [w431 _]
          tunnel: w420 -> [w430 _]
          frame True {
            n149 = invoke class="VI" method="FP.Open"(reference=w431, error in=w432, "Activate"=TRUE, "State"=w430) -> (error out=w433:errorcluster)  [unwired: 1 in, 4 out]
          }
          frame False {
          }
        }
      }
      frame "UI: Front Panel State >> Close" {
        # "Set Front Panel Open or Closed\n(Usage: \"UI: Front Panel State >> Open|Close\")"
        n150 = Unbundle By Name(w443) -> ("Core.Current VI Reference"=w442:refnum<vi>)
        n151 = property class="VI"(reference=w442, error in=w445) -> (reference out=w439:refnum<vi>, error out=w440:errorcluster, "FP.State"=w437:T4)
        n152 = Not Equal?(x=w437, y=T4."Closed" ("Front Panel Window:State")) -> (x != y?=w436:bool)
        n153 = case shown="True" w436 {
          tunnel: [w446 w449] -> w444
          tunnel: w440 -> [w446 w448]
          tunnel: w439 -> [_ w447]
          frame False {
          }
          frame True {
            n154 = invoke class="VI" method="FP.Close"(reference=w447, error in=w448) -> (error out=w449:errorcluster)  [unwired: 1 in, 2 out]
          }
        }
      }
      frame "---------- Macro ----------" {
        # "Do not put any code in this frame.\n(It is a separator no-op. You can make a copy of this frame to create a new Macro frame)"
      }
      frame "Macro: Initialize" {
        # "Initialization Macro\n(This is called once, when the VI starts)"
        n155 = Build Array (concatenate)(string[] ["Data: Initialize", "Initialize Core Data", "UI: Load Window Bounds", "Macro: Refresh UI", "UI: Initialize", "Pane: Get Properties", "UI: Show Pane Or Splitter", "UI: Front Panel State >> Open"], w455) -> (w453:string[])
      }
      frame "Macro: Refresh UI" {
        n156 = Build Array (concatenate)(string[] ["UI: Calculate Scale Factor", "UI: Get Pane And Splitter Details", "UI: Draw Nav Pic"], w460) -> (w458:string[])
      }
      frame "Macro: Exit" {
        # "Exit Macro\n(This is called once, when the VI exits)"
        n157 = Unbundle By Name(w471) -> ("Core.Close Panel on Exit?"=w470:bool)
        n158 = Select(t=string[] ["UI: Front Panel State >> Close"], s=w470, f=string[] []) -> (s? t:f=w468:string[])
        n159 = Build Array (concatenate)(w468, string[] ["UI: Save Window Bounds", "Data: Cleanup", "Exit"]) -> (w464:string[])
        n160 = Build Array (concatenate)(w464, w466) -> (w465:string[])
      }
      frame "---------- Splitter ----------" {
        # "Template Separator\n(You can make a copy of, or modify, this frame)"
      }
      frame "Splitter: Set Properties" {
        n161 = Unbundle By Name(w487) -> ("Splitters[]"=w486:refnum<class "Splitter.lvclass">[], "UI Selections.Selected Idx"=w485:i32)
        n162 = Index Array(array=w486, index=w485) -> (element=w484:refnum<class "Splitter.lvclass">)
        n163 = property class="Splitter.lvclass"(reference=w484, error in=w483, "Public Accessors:Label"="Label", "Public Accessors:Position"="Position", "Public Accessors:Sizing"="Sizing", "Public Accessors:Locked"="Locked", "Public Accessors:Color"="Color") -> (error out=w482:errorcluster)  [unwired: 1 out]
      }
      frame "Splitter: Get Properties" {
        n164 = Unbundle By Name(w499) -> ("Splitters[]"=w498:refnum<class "Splitter.lvclass">[], "UI Selections.Selected Idx"=w497:i32)
        n165 = Index Array(array=w498, index=w497) -> (element=w496:refnum<class "Splitter.lvclass">)
        n166 = property class="Splitter.lvclass"(reference=w496, error in=w495) -> (error out=w494:errorcluster, "Public Accessors:Label"=w493:string, "Public Accessors:Position"=w492:i32, "Public Accessors:Sizing"=w491:T1, "Public Accessors:Locked"=w490:bool, "Public Accessors:Color"=w489:u32)  [unwired: 1 out]
        n167 = local write "Label"(w493) -> ()
        n168 = local write "Position"(w492) -> ()
        n169 = local write "Sizing"(w491) -> ()
        n170 = local write "Locked"(w490) -> ()
        n171 = local write "Color"(w489) -> ()
      }
      frame "---------- Pane ----------" {
        # "Template Separator\n(You can make a copy of, or modify, this frame)"
      }
      frame "Pane: Set Properties" {
        n172 = Unbundle By Name(w515) -> ("Panes[]"=w514:refnum<class "Pane.lvclass">[], "UI Selections.Selected Idx"=w513:i32)
        n173 = local read "Color"() -> (w504:u32)
        n174 = local read "Label"() -> (w505:string)
        n175 = Index Array(array=w514, index=w513) -> (element=w512:refnum<class "Pane.lvclass">)
        n176 = property class="Pane.lvclass"(reference=w512, error in=w511, "Public Accessors:Label"=w505, "Public Accessors:Min Pane Size"="Min Pane Size", "Public Accessors:Origin"="Origin", "Public Accessors:Horizontal Scroll"="Horizontal Scroll", "Public Accessors:Vertical Scroll"="Vertical Scroll", "Public Accessors:Color"=w504) -> (error out=w510:errorcluster)  [unwired: 1 out]
      }
      frame "Pane: Get Properties" {
        n177 = Unbundle By Name(w528) -> ("Panes[]"=w527:refnum<class "Pane.lvclass">[], "UI Selections.Selected Idx"=w526:i32)
        n178 = Index Array(array=w527, index=w526) -> (element=w525:refnum<class "Pane.lvclass">)
        n179 = property class="Pane.lvclass"(reference=w525, error in=w524) -> (error out=w523:errorcluster, "Public Accessors:Label"=w522:string, "Public Accessors:Min Pane Size"=w521:T3, "Public Accessors:Origin"=w520:T3, "Public Accessors:Horizontal Scroll"=w519:T2, "Public Accessors:Vertical Scroll"=w518:T2, "Public Accessors:Color"=w517:u32)  [unwired: 1 out]
        n180 = local write "Label"(w522) -> ()
        n181 = local write "Min Pane Size"(w521) -> ()
        n182 = local write "Origin"(w520) -> ()
        n183 = local write "Horizontal Scroll"(w519) -> ()
        n184 = local write "Vertical Scroll"(w518) -> ()
        n185 = local write "Color"(w517) -> ()
      }
    }
  }
  "Error Out" <- w2
